vi "test-Function-Generator-Test1.vi"(8 "error in (no error)":errorcluster) -> (0 "error out":errorcluster, 3 "All tests passed":bool)   [LabVIEW 2019]
uses:
  <vilib>/Rock Robotics/WPI/ThirdParty/JAS_Junk/TrajLib/X_Y_PAIR.ctl
  <vilib>/Rock Robotics/WPI/ThirdParty/JAS_Junk/TrajLib/FunctionGenerator_Add_Value.vi
  <vilib>/gmath/interp.llb/Search Ordered Table.vi
  <vilib>/Rock Robotics/WPI/ThirdParty/JAS_Junk/TrajLib/Trajectory_Library.lvlib
panel:
  out "Output T 6":dbl
  out "Output T 5":dbl
  out "Output T 4":dbl
  out "Output T 3":dbl
  out "Table Ys":dbl[](array[numeric])
  out "Table Xs":dbl[](array[numeric])
  out "Output T 2":dbl
  out "Output T 1":dbl
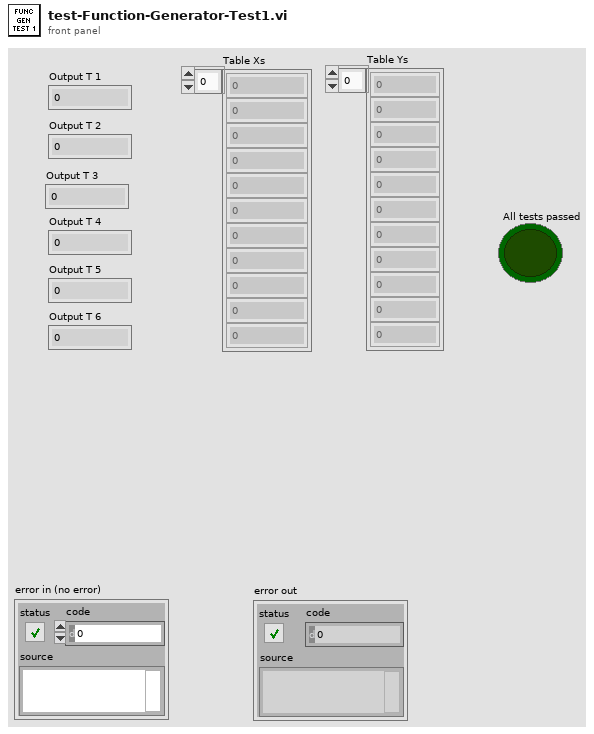
[diagram p1: front panel]
types:
  T1 = typedef "Trajectory_Library.lvlib/X_Y_PAIR.ctl" = cluster{"X":dbl, "Y":dbl}
  T2 = typedef "Trajectory_Library.lvlib/FUNCTION_GENERATOR.ctl" = cluster{"Table Xs":dbl[], "Table Ys":dbl[], "MinX":dbl, "MaxX":dbl, "ItemCount":i32}
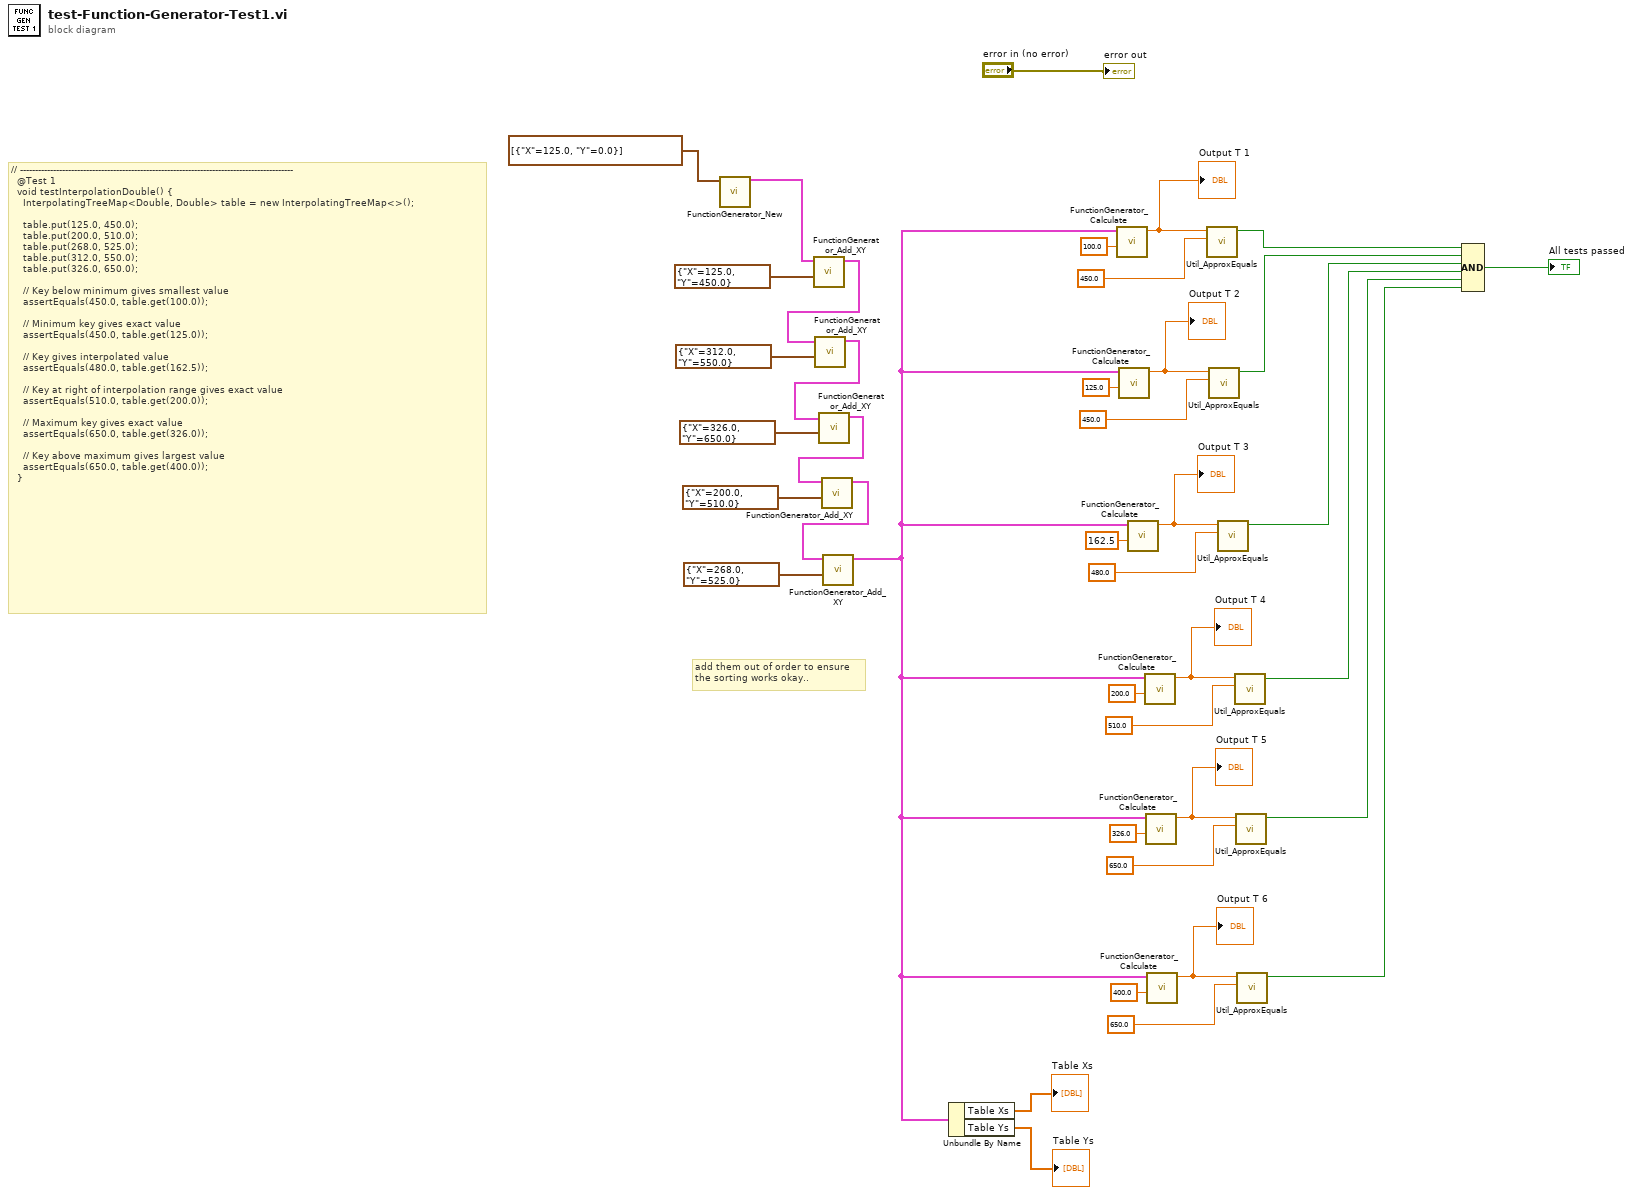
[diagram p0: block diagram]
diagram:
  # "add them out of order to ensure\nthe sorting works okay.."
  # "// -------------------------------------------------------------------------------------------\n  @Test 1\n  void testInterpolationDouble() {\n    InterpolatingTreeMap<Double, Double> table = new InterpolatingTreeMap<>();\n\n    table.put(125.0, 450.0);\n    table.put(200.0, 510.0);\n    table.put(268.0, 525.0);\n    table.put(312.0, 550.0);\n    table.put(326.0, 650.0);\n\n    // Key below minimum gives smallest value\n    assertEquals(450.0, table.get(100.0));\n\n    // Minimum key gives exact value\n    assertEquals(450.0, table.get(125.0));\n\n    // Key gives interpolated value\n    assertEquals(480.0, table.get(162.5));\n\n    // Key at right of interpolation range gives exact value\n    assertEquals(510.0, table.get(200.0));\n\n    // Maximum key gives exact value\n    assertEquals(650.0, table.get(326.0));\n\n    // Key above maximum gives largest value\n    assertEquals(650.0, table.get(400.0));\n  }"
  n1 = call <vilib>:"FunctionGenerator_New.vi"("X Y Pairs"=T1[] [{"X"=125.0, "Y"=0.0}]) -> ("FUNCTION_GENERATOR"=w18:T2)  [unwired: 10 in]
  n2 = call <vilib>:"FunctionGenerator_Add_XY.vi"("X_Y_PAIR"=T1 {"X"=125.0, "Y"=450.0}, "in FUNCTION_GENERATOR"=w18) -> ("out FUNCTION_GENERATOR"=w33:T2)  [unwired: 9 in]
  n3 = call <vilib>:"FunctionGenerator_Add_XY.vi"("X_Y_PAIR"=T1 {"X"=312.0, "Y"=550.0}, "in FUNCTION_GENERATOR"=w33) -> ("out FUNCTION_GENERATOR"=w32:T2)  [unwired: 9 in]
  n4 = call <vilib>:"FunctionGenerator_Add_XY.vi"("X_Y_PAIR"=T1 {"X"=326.0, "Y"=650.0}, "in FUNCTION_GENERATOR"=w32) -> ("out FUNCTION_GENERATOR"=w31:T2)  [unwired: 9 in]
  n5 = call <vilib>:"FunctionGenerator_Add_XY.vi"("X_Y_PAIR"=T1 {"X"=200.0, "Y"=510.0}, "in FUNCTION_GENERATOR"=w31) -> ("out FUNCTION_GENERATOR"=w30:T2)  [unwired: 9 in]
  n6 = call <vilib>:"FunctionGenerator_Add_XY.vi"("X_Y_PAIR"=T1 {"X"=268.0, "Y"=525.0}, "in FUNCTION_GENERATOR"=w30) -> ("out FUNCTION_GENERATOR"=w3:T2)  [unwired: 9 in]
  n7 = Unbundle By Name(w3) -> ("Table Xs"=→"Table Xs":dbl[], "Table Ys"=→"Table Ys":dbl[])
  n8 = call <vilib>:"FunctionGenerator_Calculate.vi"("Input Value"=100.0, "FUNCTION_GENERATOR"=w3) -> ("Output Value"=w28:dbl)  [unwired: 9 in]
  "Output T 1" <- w28
  n9 = call <vilib>:"FunctionGenerator_Calculate.vi"("Input Value"=125.0, "FUNCTION_GENERATOR"=w3) -> ("Output Value"=w21:dbl)  [unwired: 9 in]
  "Output T 2" <- w21
  n10 = call <vilib>:"FunctionGenerator_Calculate.vi"("Input Value"=162.5, "FUNCTION_GENERATOR"=w3) -> ("Output Value"=w15:dbl)  [unwired: 9 in]
  "Output T 3" <- w15
  n11 = call <vilib>:"FunctionGenerator_Calculate.vi"("Input Value"=200.0, "FUNCTION_GENERATOR"=w3) -> ("Output Value"=w12:dbl)  [unwired: 9 in]
  "Output T 4" <- w12
  n12 = call <vilib>:"FunctionGenerator_Calculate.vi"("Input Value"=326.0, "FUNCTION_GENERATOR"=w3) -> ("Output Value"=w7:dbl)  [unwired: 9 in]
  "Output T 5" <- w7
  n13 = call <vilib>:"FunctionGenerator_Calculate.vi"("Input Value"=400.0, "FUNCTION_GENERATOR"=w3) -> ("Output Value"=w4:dbl)  [unwired: 9 in]
  "Output T 6" <- w4
  n14 = call <vilib>:"Util_ApproxEquals.vi"("Value 2"=450.0, "Value 1"=w28) -> ("ApproxEquals"=w26:bool)  [unwired: 9 in]
  n15 = call <vilib>:"Util_ApproxEquals.vi"("Value 2"=450.0, "Value 1"=w21) -> ("ApproxEquals"=w22:bool)  [unwired: 9 in]
  n16 = call <vilib>:"Util_ApproxEquals.vi"("Value 2"=480.0, "Value 1"=w15) -> ("ApproxEquals"=w11:bool)  [unwired: 9 in]
  n17 = call <vilib>:"Util_ApproxEquals.vi"("Value 2"=510.0, "Value 1"=w12) -> ("ApproxEquals"=w10:bool)  [unwired: 9 in]
  n18 = call <vilib>:"Util_ApproxEquals.vi"("Value 2"=650.0, "Value 1"=w7) -> ("ApproxEquals"=w2:bool)  [unwired: 9 in]
  n19 = call <vilib>:"Util_ApproxEquals.vi"("Value 2"=650.0, "Value 1"=w4) -> ("ApproxEquals"=w1:bool)  [unwired: 9 in]
  n20 = Compound Arithmetic op=AND(w26, w22, w11, w10, w2, w1) -> (→"All tests passed":bool)
  "error out" <- "error in (no error)"
